vi "heron-use-test.vi"() -> ()   [LabVIEW 2024]
panel:
  in  "c":dbl
  in  "b":dbl
  in  "a":dbl
  out "Area":dbl
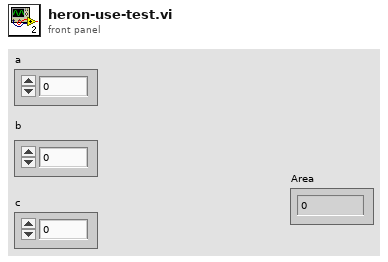
[diagram p1: front panel]
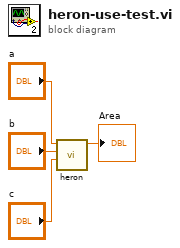
[diagram p0: block diagram]
diagram:
  n1 = call "heron.vi"("c"="c", "b"="b", "a"="a") -> ("area"=→"Area":dbl)  [unwired: 8 in]
